vi "PlanPath.vi"() -> ()   [LabVIEW 2016]
uses:
  <vilib>/Utility/file.llb/Read Delimited Spreadsheet (DBL).vi
panel:
  in  "Position data":T1
  in  "Ref_point":cluster{"Lat":dbl, "Long":dbl}
  out "Delta Heading":dbl
  out "all rows":dbl[][](array[numeric])
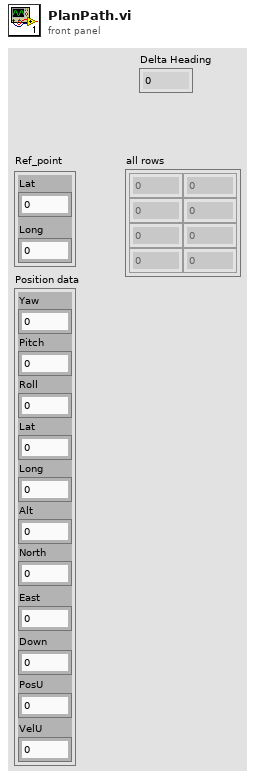
[diagram p1: front panel]
types:
  T1 = cluster{"Alt":dbl, "Long":dbl, "Lat":dbl, "Roll":sgl, "Pitch":sgl, "Yaw":sgl, "North":dbl, "East":dbl, "Down":dbl, "PosU":dbl, "VelU":dbl}
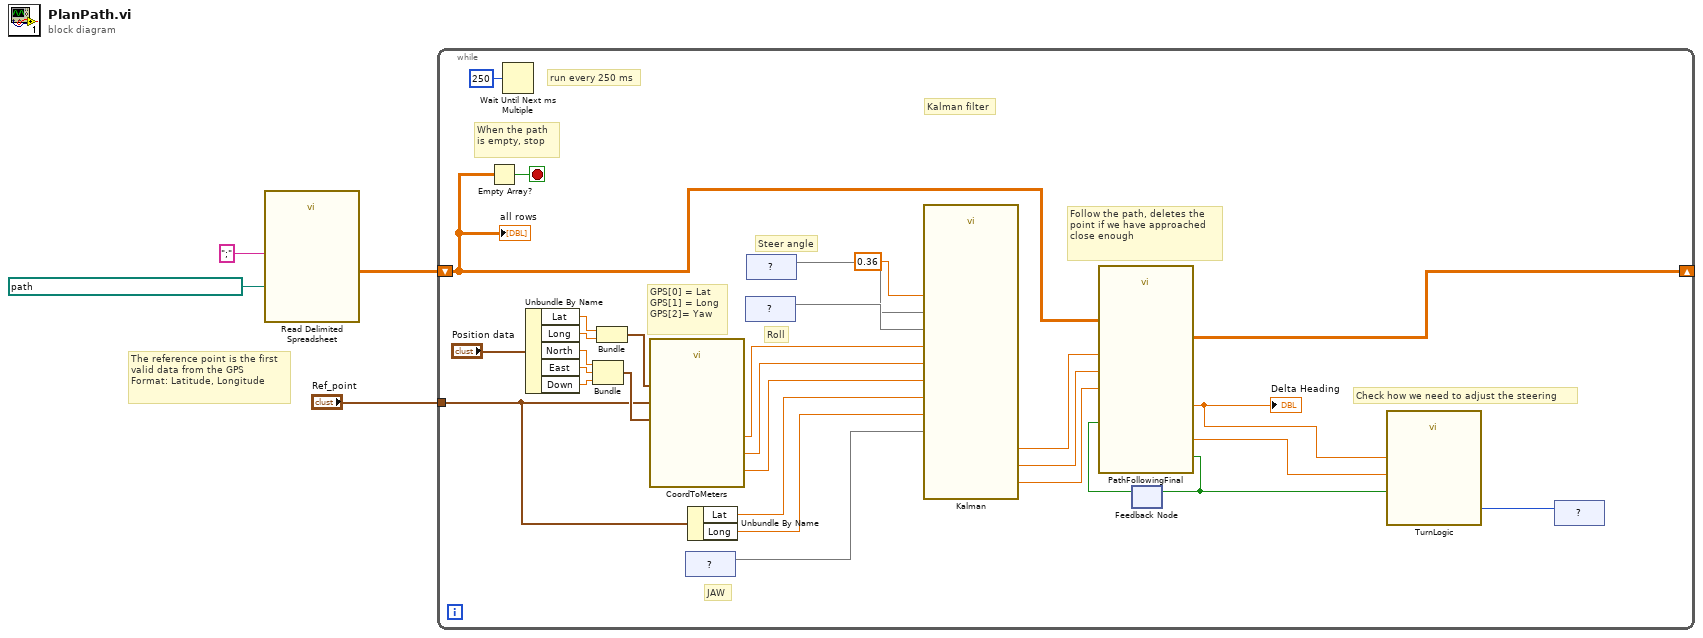
[diagram p0: block diagram]
diagram:
  # "The reference point is the first valid data from the GPS\nFormat: Latitude, Longitude"
  n1 = call-poly <vilib>:"Read Delimited Spreadsheet.vi"("file path (dialog if empty)"=path "C:/Users/Starmachine24/Desktop/tänk.txt", "delimiter (\\t)"=";" ("delimiter (\\t)")) -> ("all rows"=w2:dbl[][])  [unwired: 8 in, 5 out]
  n2 = while {
    shift-right: [w32] -> _
    shift-left: w2 -> [w18]
    tunnel: "Ref_point" -> [w8]
    stop <- w33 stop-if-true
    # "Roll"
    # "Steer angle"
    # "JAW"
    # "Check how we need to adjust the steering"
    # "Kalman filter"
    # "run every 250 ms"
    # "Follow the path, deletes the point if we have approached close enough"
    # "GPS[0] = Lat\nGPS[1] = Long \nGPS[2]= Yaw"
    # "When the path is empty, stop"
    n3 = Empty Array?(array=w18) -> (empty?=w33:bool)
    n4 = Wait Until Next ms Multiple(millisecond multiple=u32 250) -> ()  [unwired: 1 out]
    n5 = Unbundle By Name("Position data") -> ("Lat"=w25:dbl, "Long"=w24:dbl, "North"=w22:dbl, "East"=w21:dbl, "Down"=w20:dbl)
    n6 = Bundle("North"=w22, "East"=w21, "Down"=w20) -> (w19:cluster{"North":dbl, "East":dbl, "Down":dbl})  [unwired: 1 in]
    n7 = Bundle("Lat"=w25, "Long"=w24) -> (w23:cluster{"Lat":dbl, "Long":dbl})  [unwired: 1 in]
    n8 = call "CoordToMeters.vi"("VelNed"=w19, "Ref Point"=w8, "GPS position"=w23) -> ("Bike Heading"=w15:dbl, "X"=w16:dbl, "Y"=w17:dbl)  [unwired: 6 in]
    n9 = shared-variable "?"() -> (w5)  [unwired: 1 in, 1 out]
    n10 = Unbundle By Name(w8) -> ("Lat"=w7:dbl, "Long"=w6:dbl)
    n11 = shared-variable "?"() -> (w10)  [unwired: 1 in, 1 out]
    n12 = shared-variable "?"() -> (w9)  [unwired: 1 in, 1 out]
    n13 = call "Kalman.vi"("x"=w6, "y"=w7, "theta"=w5, "GPS X"=w16, "GPS Y"=w17, "GPS theta"=w15, "ds"=0.36, "phi"=w10, "delta"=w9) -> ("new x"=w12:dbl, "new y"=w13:dbl, "new theta"=w11:dbl)  [unwired: 8 in]
    n14 = feedback #1() -> (w31:bool)  [unwired: 1 in]
    n15 = call "PathFollowingFinal.vi"("GPS_Lat"=w13, "GPS_Long"=w12, "Path"=w18, "Heading angle"=w11, "Save heading"=w31) -> ("Path rest"=w32:dbl[][], "Delta Heading Angle"=w29:dbl, "Goal reached"=w28:bool, "Beta"=w30:dbl)  [unwired: 7 in]
    "Delta Heading" <- w29
    n16 = feedback-in #1(w28) -> ()
    n17 = call "TurnLogic.vi"("Goal Reached"=w28, "Beta"=w30, "Delta Theta"=w29) -> ("Increment Lean"=w27:i8)  [unwired: 8 in]
    n18 = shared-variable "?"(w27) -> ()  [unwired: 1 in, 1 out]
    "all rows" <- w18
  }
